vi "Main.vi"() -> ()   [LabVIEW 2025]
uses:
  Controls/StopGlobal.vi
panel:
  in  "AlreadyChangeToGame":bool
  out "reference out":refnum<vi>
  in  "stop":bool
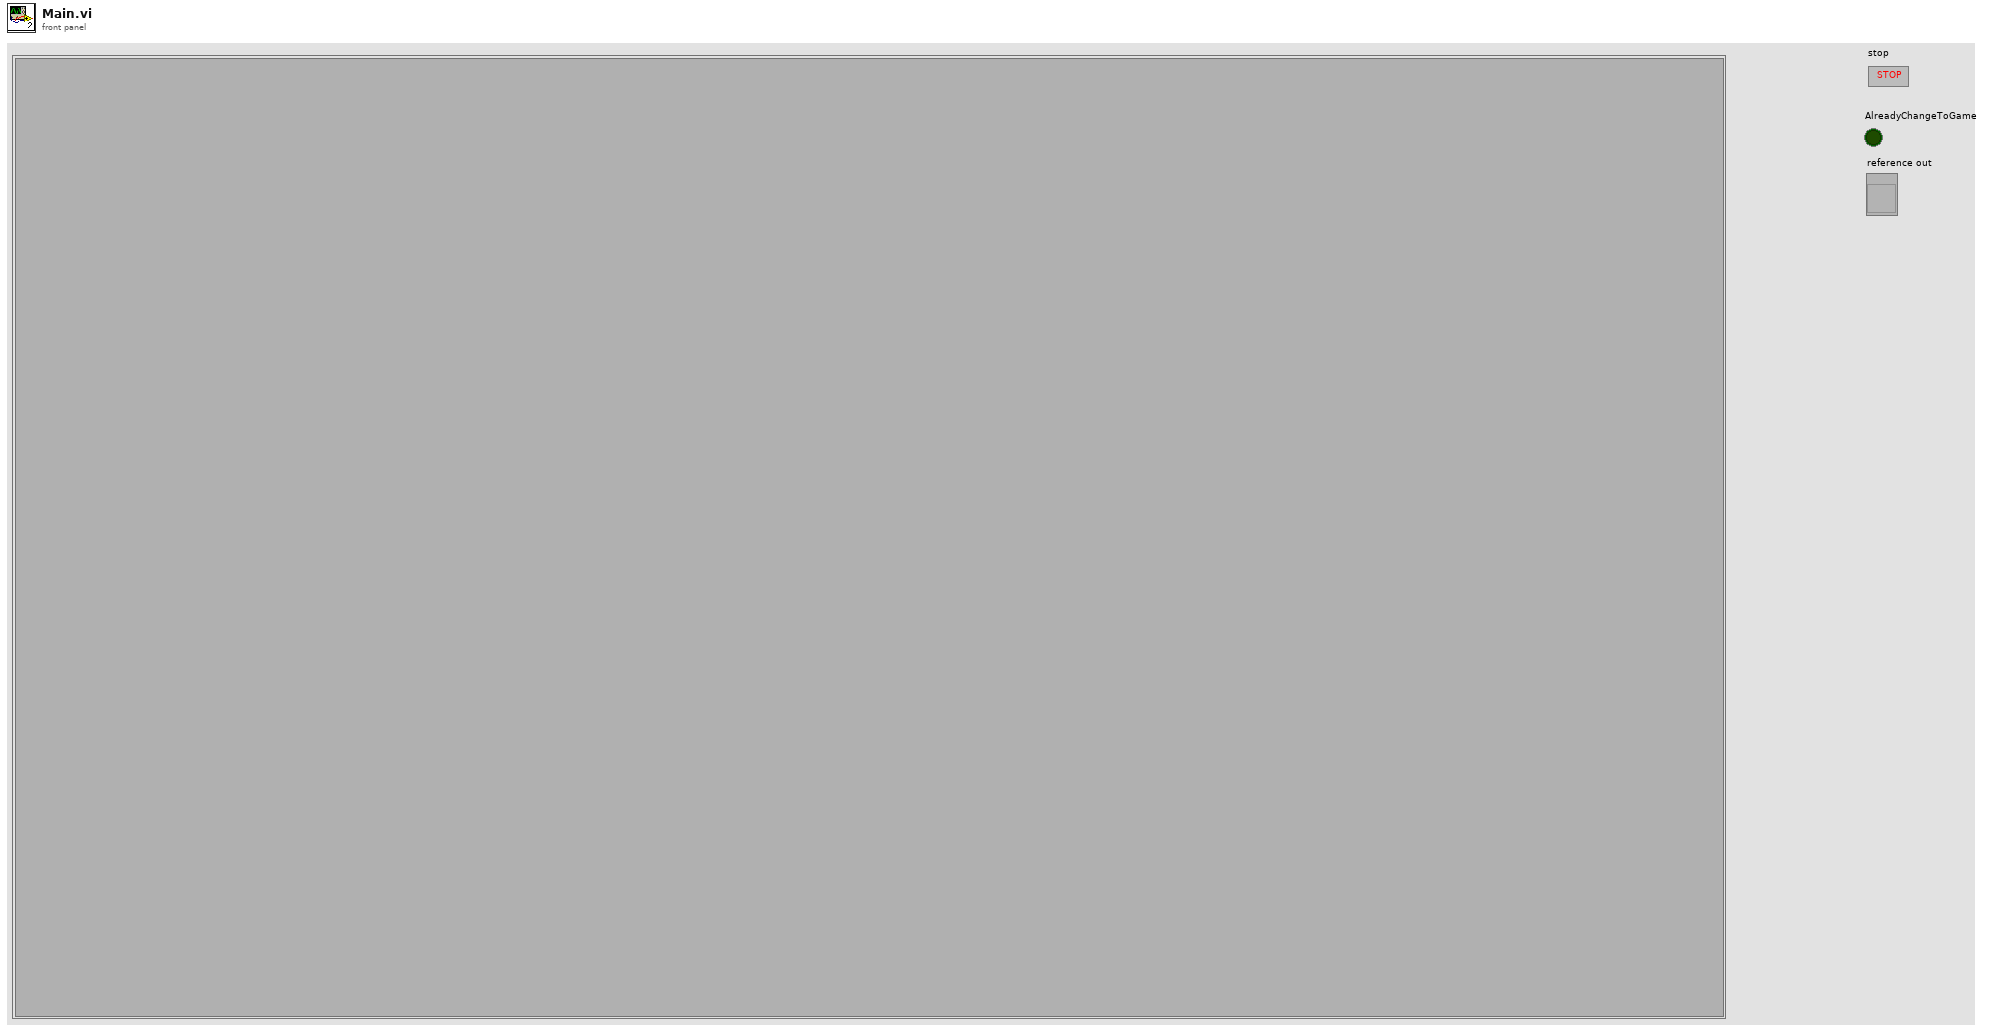
[diagram p1: front panel]
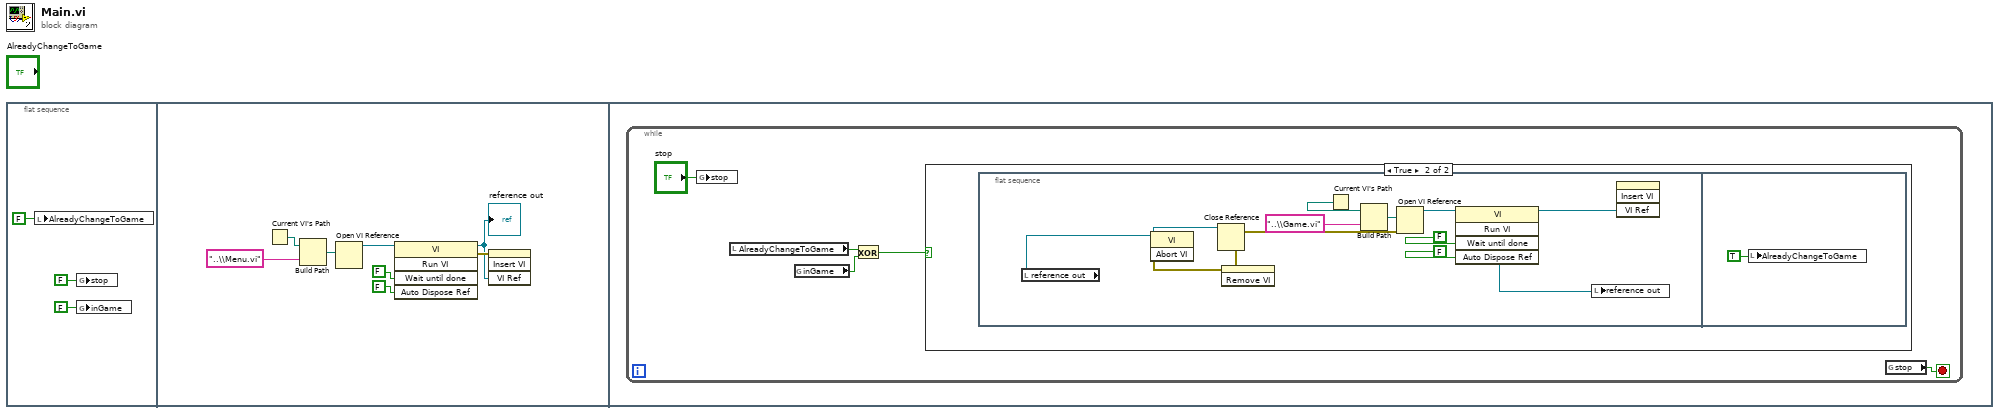
[diagram p0: block diagram]
diagram:
  n1 = flat-sequence {
    frame #0 {
      n2 = local write "AlreadyChangeToGame"(FALSE) -> ()
      n3 = global write "StopGlobal.vi" "stop"(FALSE) -> ()
      n4 = global write "StopGlobal.vi" "inGame"(FALSE) -> ()
    }
    frame #1 {
      n5 = Current VI's Path() -> (path=w7:path)
      n6 = Build Path(base path=w7, name or relative path="..\\Menu.vi") -> (appended path=w8:path)
      n7 = Open VI Reference(vi path=w8) -> (vi reference=w9:refnum<vi>)  [unwired: 5 in, 1 out]
      n8 = invoke class="VI" method="Run VI"(reference=w9, "Wait until done"=FALSE ("Wait Until Done"), "Auto Dispose Ref"=FALSE ("Auto Dispose Reference")) -> (reference out=w10:refnum<vi>, error out=w11:errorcluster)  [unwired: 2 in, 3 out]
      "reference out" <- w10
      n9 = invoke class="SubPnl" method="Insert VI"(error in=w11, "VI Ref"=w10) -> ()  [unwired: 2 in, 4 out]
    }
    frame #2 {
      n10 = while {
        stop <- w16 stop-if-true
        n11 = global write "StopGlobal.vi" "stop"("stop") -> ()
        n12 = local read "AlreadyChangeToGame"() -> (w13:bool)
        n13 = global read "StopGlobal.vi" "inGame"() -> (w14:bool)
        n14 = Exclusive Or(1:w14, 2:w13) -> (0:w12:bool)
        n15 = case shown="True" w12 {
          frame False {
          }
          frame True {
            n16 = flat-sequence {
              frame #0 {
                n17 = local read "reference out"() -> (w25:refnum<vi>)
                n18 = invoke class="VI" method="Abort VI"(reference=w25) -> (reference out=w26:refnum<vi>, error out=w27:errorcluster)  [unwired: 2 in, 1 out]
                n19 = Close Reference(reference=w26) -> ()  [unwired: 1 in, 1 out]
                n20 = invoke class="SubPnl" method="Remove VI"(error in=w27) -> (error out=w17:errorcluster)  [unwired: 2 in, 2 out]
                n21 = Current VI's Path() -> (path=w21:path)
                n22 = Build Path(base path=w21, name or relative path="..\\Game.vi") -> (appended path=w23:path)
                n23 = Open VI Reference(vi path=w23, error in (no error)=w17) -> (vi reference=w24:refnum<vi>)  [unwired: 4 in, 1 out]
                n24 = invoke class="VI" method="Run VI"(reference=w24, "Wait until done"=FALSE ("Wait Until Done"), "Auto Dispose Ref"=FALSE ("Auto Dispose Reference")) -> (reference out=w22:refnum<vi>)  [unwired: 2 in, 4 out]
                n25 = local write "reference out"(w22) -> ()
                n26 = invoke class="SubPnl" method="Insert VI"("VI Ref"=w22) -> ()  [unwired: 3 in, 4 out]
              }
              frame #1 {
                n27 = local write "AlreadyChangeToGame"(TRUE ("AlreadyChangeToGame")) -> ()
              }
            }
          }
        }
        n28 = global read "StopGlobal.vi" "stop"() -> (w16:bool)
      }
    }
  }
